vi "GetGlobalVariable.vi"   [LabVIEW 2010]
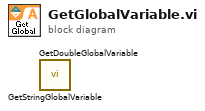
[diagram p0: block diagram]
diagram:
  n1 = call "GetStringGlobalVariable.vi"() -> ()  [unwired: 9 in, 3 out]
  n2 = call "GetDoubleGlobalVariable.vi"() -> ()  [unwired: 9 in, 3 out]
